vi "SetWindowActive.vi"(8 "Error In":errorcluster, 11 "Window Name":string) -> (0 "Error Out":errorcluster)   [LabVIEW 2016, in "DronaTest.lvlib"]
doc: "This VI will programmatically move a window to the front whether its a LabVIEW window or not."
uses:
  DronaTest.lvlib
  C:/Windows/System32/user32.dll
panel:
  out "Error":i32
  out "Handle":dbl
  # "Overview: This VI will programmatically move a window to the front whether its a LabVIEW window or not.\nRequirements: LabVIEW 2012 (or compatible)\nInstructions: \n1. Choose the window name you want to bring to front\n2. Run the VI\n3. Stop Execution"
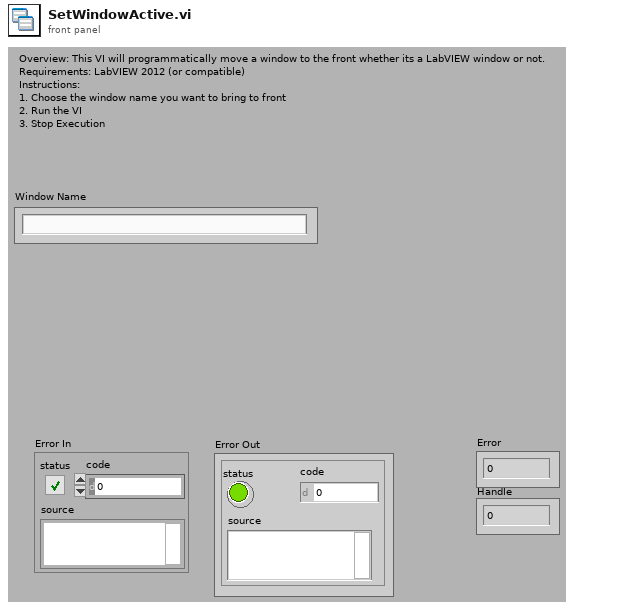
[diagram p1: front panel]
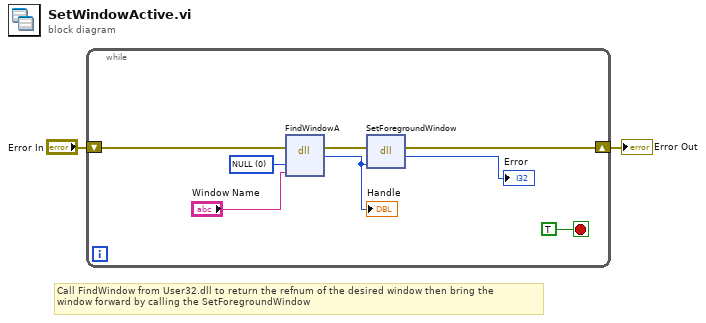
[diagram p0: block diagram]
diagram:
  # "Call FindWindow from User32.dll to return the refnum of the desired window then bring the \nwindow forward by calling the SetForegroundWindow"
  n1 = while {
    shift-right: [w10] -> w2
    shift-left: "Error In" -> [w9]
    stop <- TRUE stop-if-true
    w8 = 0 items=["NULL"]
    n2 = dll-call lib="C:/Windows/System32/user32.dll" fn="FindWindowA" label="FindWindow"(error in=w9, "lpszClassName"=w8, "lpszWindowName"="Window Name") -> (error out=w4:errorcluster, "hWnd"=w6:u32)  [unwired: 3 in, 2 out]
    "Handle" <- w6
    n3 = dll-call lib="C:/Windows/System32/user32.dll" fn="SetForegroundWindow"(error in=w4, "Handle"=w6) -> (error out=w10:errorcluster, "return type"=→"Error":i32)  [unwired: 3 in, 1 out]
  }
  "Error Out" <- w2
